vi "Teleop Shooter Control.vi"(8 "Manipulator D-Pad":T2, 9 "Manipulator Buttons":T3, 10 "Driver Buttons":T3, 11 "Manipulator Axes":T1) -> ()   [LabVIEW 2015]
uses:
  Common Code/Gamepads/Button Cluster.ctl
  Common Code/Gamepads/D-Pad.ctl
  Common Code/Gamepads/Axes Cluster.ctl
  Common Code/Shooter Commands.ctl
  Common Code/Change Detect.vi
  Common Code/Change Detect Boolean.vi
  Robot Global Data.vi
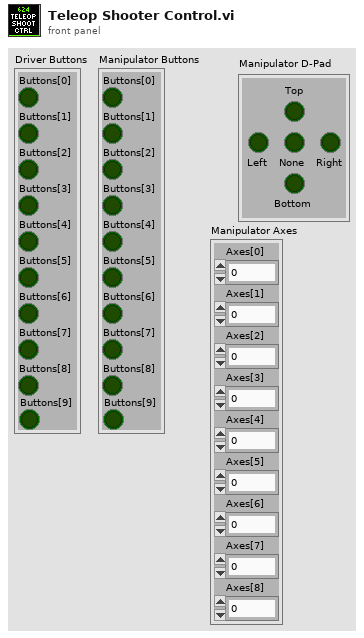
[diagram p1: front panel]
types:
  T1 = typedef "Axes Cluster.ctl" = cluster{"Axes[0]":dbl, "Axes[1]":dbl, "Axes[2]":dbl, "Axes[3]":dbl, "Axes[4]":dbl, "Axes[5]":dbl, "Axes[6]":dbl, "Axes[7]":dbl, "Axes[8]":dbl}
  T2 = typedef "D-Pad.ctl" = cluster{"Top":bool, "Bottom":bool, "None":bool, "Right":bool, "Left":bool}
  T3 = typedef "Button Cluster.ctl" = cluster{"Buttons[0]":bool, "Buttons[1]":bool, "Buttons[2]":bool, "Buttons[3]":bool, "Buttons[4]":bool, "Buttons[5]":bool, "Buttons[6]":bool, "Buttons[7]":bool, "Buttons[8]":bool, "Buttons[9]":bool}
  T4 = enum16{"0", "1", "2", "3", "4", "5", "6", "7", "8", "9", "A", "B", "C", "D", "E", "F", "G", "H", "I", "J", "K", "L", "M", "N", "O", "P", "Q", "R", "S", "T", "U", "V", "W", "X", "Y", "Z", "F1", "F2", "F3", "F4", "F5", "F6", "F7", "F8", "F9", "F10", "F11", "F12", "F13", "F14", "F15", "ADD", "BACK", "BACKSLASH", "CAPITAL", "COMMA", "DECIMAL", "DELETE", "DIVIDE", "DOWN", "END", "EQUALS", "ESCAPE", "GRAVE (`)", "HOME", "INSERT", "LBRACKET", "LCONTROL", "LEFT", "L ALT", "LSHIFT", "LWIN", "MINUS", "MULTIPLY", "NEXT", "NUMLOCK", "NUMPAD_0", "NUMPAD_1", "NUMPAD_2", "NUMPAD_3", "NUMPAD_4", "NUMPAD_5", "NUMPAD_6", "NUMPAD_7", "NUMPAD_8", "NUMPAD_9", "PAUSE", "PERIOD", "PRIOR (PG UP)", "RBRACKET", "RCONTROL", "RETURN", "RIGHT", "R ALT", "RSHIFT", "RWIN", "SCROLL", "SEMICOLON", "SLASH", "SPACE", "SUBTRACT", "TAB", "UP", "ENTER (num pad)", "' (quote)"}
  T5 = typedef "Shoot Modes Enum.ctl" = enum16{"Manual", "Safe", "Auto"}
  T6 = typedef "Shooter Commands.ctl" = enum16{"Idle", "Prime Shooter", "Shoot"}
  T7 = typedef "Shot Type.ctl" = enum16{"Batter Shot", "Corner Shot", "Curve Shot", "Vision Shot", "Deep Middle Shot"}
  T8 = typedef "Manual Shoot.ctl" = cluster{"Spin Wheels":bool, "Fire":bool, "Angle":dbl, "Angle Power":dbl, "Use Manual Angle":bool, "Override RPM":bool, "Left RPM":dbl, "Right RPM":dbl, "Secure Ball?":bool}
  T9 = typedef "Shooter Command Cluster.ctl" = cluster{"Command":T6, "Mode":T5, "Shot Type":T7, "Override Trigger IR":bool, "Override Angle?":bool}
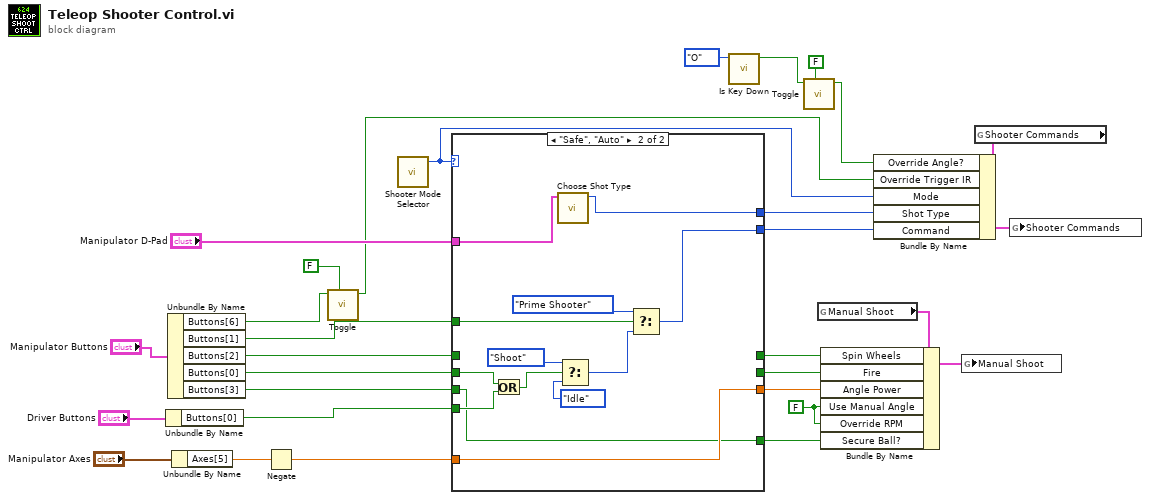
[diagram p0: block diagram]
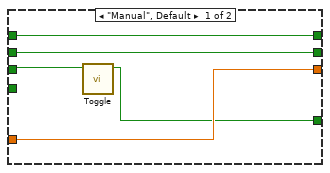
[diagram p2: hidden frame]
diagram:
  w7 = FALSE ("Use Manual Angle")
  n1 = Unbundle By Name("Driver Buttons") -> ("Buttons[0]"=w16:bool)
  n2 = Unbundle By Name("Manipulator Buttons") -> ("Buttons[6]"=w10:bool, "Buttons[1]"=w28:bool, "Buttons[2]"=w25:bool, "Buttons[0]"=w18:bool, "Buttons[3]"=w6:bool)
  n3 = Unbundle By Name("Manipulator Axes") -> ("Axes[5]"=w14:dbl)
  n4 = Negate(x=w14) -> (-x=w12:dbl)
  n5 = call "Toggle.vi"("Initial Value"=FALSE, "In"=w10) -> ("Toggled"=w9:bool)  [unwired: 9 in]
  n6 = call "Shooter Mode Selector.vi"() -> ("Mode"=w11:T5)  [unwired: 11 in]
  n7 = case shown="\"Safe\", \"Auto\"" w11 {
    tunnel: w28 -> [_ w44]
    tunnel: [_ w47] -> w27
    tunnel: w25 -> [w35 _]
    tunnel: [w35 _] -> w23
    tunnel: [w33 _] -> w21
    tunnel: "Manipulator D-Pad" -> [_ w46]
    tunnel: [_ w45] -> w19
    tunnel: w18 -> [w33 w40]
    tunnel: w16 -> [_ w39]
    tunnel: [w34 w37] -> w13
    tunnel: w12 -> [w34 w37]
    tunnel: w6 -> [w32 w36]
    tunnel: [w31 w36] -> w5
    frame "Manual", Default {
      n8 = call "Toggle.vi"("In"=w32) -> ("Toggled"=w31:bool)  [unwired: 10 in]
    }
    frame "Safe", "Auto" {
      n9 = Or(x=w40, y=w39) -> (x .or. y?=w38:bool)
      n10 = call "Choose Shot Type.vi"("Manipulator D-Pad"=w46) -> ("Shot Type"=w45:T7)  [unwired: 10 in]
      n11 = Select(t=Shooter_Commands."Shoot", s=w38, f=Shooter_Commands."Idle" ("Command")) -> (s? t:f=w41:T6)
      n12 = Select(t=Shooter_Commands."Prime Shooter" ("Command"), s=w44, f=w41) -> (s? t:f=w47:T6)
    }
  }
  n13 = call "Is Key Down.vi"("Key"=T4."O") -> ("Key Down?"=w4:bool)  [unwired: 10 in]
  n14 = call "Toggle.vi"("Initial Value"=FALSE, "In"=w4) -> ("Toggled"=w3:bool)  [unwired: 9 in]
  n15 = global read "Robot Global Data.vi" "Manual Shoot"() -> (w24:T8)
  n16 = Bundle By Name(cluster=w24, "Spin Wheels"=w23, "Fire"=w21, "Angle Power"=w13, "Use Manual Angle"=w7, "Override RPM"=w7, "Secure Ball?"=w5) -> (w22:T8)
  n17 = global write "Robot Global Data.vi" "Manual Shoot"(w22) -> ()
  n18 = global read "Robot Global Data.vi" "Shooter Commands"() -> (w26:T9)
  n19 = Bundle By Name(cluster=w26, "Override Angle?"=w3, "Override Trigger IR"=w9, "Mode"=w11, "Shot Type"=w19, "Command"=w27) -> (w29:T9)
  n20 = global write "Robot Global Data.vi" "Shooter Commands"(w29) -> ()
